vi "Add bindings (SubVI).vi"(2 "error in (no error)":errorcluster, 3 "binding key":string[](array[string]), 4 "Exchange.lvclass":refnum<class "Exchange.lvclass">, 5 "Queue in":refnum<class "Queue.lvclass">) -> (0 "error out":errorcluster, 1 "Queue out":refnum<class "Queue.lvclass">)   [LabVIEW 2016]
uses:
  <vilib>/Distrio/LabbitMQ/Exchange/Exchange.lvclass
  <vilib>/Distrio/LabbitMQ/Queue/Queue.lvclass
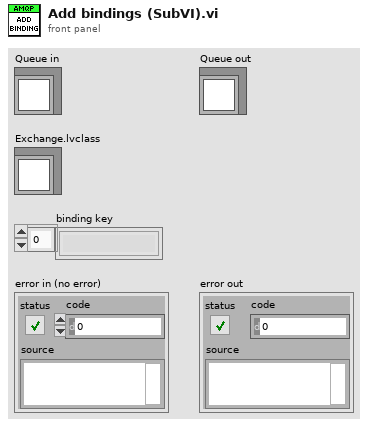
[diagram p1: front panel]
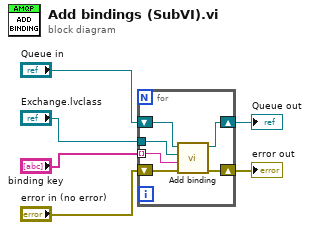
[diagram p0: block diagram]
diagram:
  n1 = for {
    tunnel: "binding key" -> [w11] mode=indexing
    shift-right: [w10] -> w3
    shift-left: "Queue in" -> [w12]
    shift-right: [w9] -> w4
    shift-left: "error in (no error)" -> [w8]
    tunnel: "Exchange.lvclass" -> [w7]
    n2 = call <vilib>:"Add binding.vi"("error in (no error)"=w8, "binding key"=w11, "Exchange.lvclass"=w7, "Consumer in"=w12) -> ("error out"=w9:errorcluster, "Consumer out"=w10:refnum<class "Queue.lvclass">)  [unwired: 6 in]
  }
  "error out" <- w4
  "Queue out" <- w3
